vi "lpf.vi"(1 "Signals":waveform(dbl)[](array[waveform])) -> (0 "FIltered signals":waveform(dbl)[](array[waveform]))   [LabVIEW 2021]
uses:
  <vilib>/Analysis/3filter.llb/Filter Passband Type.ctl
  <vilib>/Analysis/3filter.llb/Butterworth Filter (DBL).vi
  <vilib>/Analysis/NI_AALBase.lvlib
panel:
  in  "Cutoff frequency, Hz":dbl=100.0
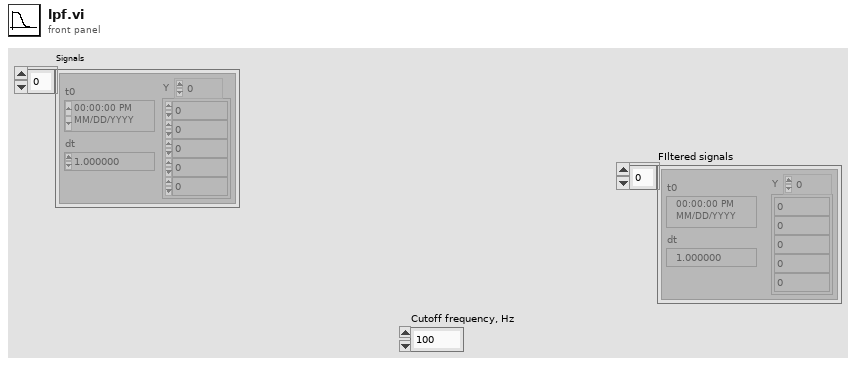
[diagram p1: front panel]
types:
  T1 = typedef "NI_AALBase.lvlib/Filter Passband Type.ctl" = enum32{"Lowpass", "Highpass", "Bandpass", "Bandstop"}
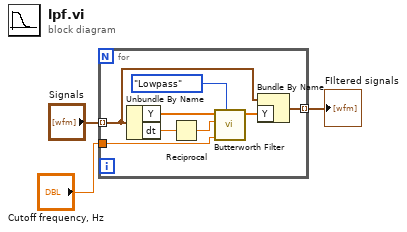
[diagram p0: block diagram]
diagram:
  n1 = for {
    tunnel: "Signals" -> [w6] mode=indexing
    tunnel: "Cutoff frequency, Hz" -> [w7]
    tunnel: [w4] -> w1 mode=indexing
    n2 = Unbundle By Name(w6) -> ("Y"=w11:dbl[], "dt"=w10:dbl)
    n3 = Reciprocal(x=w10) -> (1/x=w9:dbl)
    n4 = call-poly <vilib>:"Butterworth Filter.vi"("filter type"=Filter_Passband_Type."Lowpass", "low cutoff freq: fl"=w7, "sampling freq: fs"=w9, "X"=w11) -> ("Filtered X"=w5:dbl[])  [unwired: 4 in, 1 out]
    n5 = Bundle By Name(cluster=w6, "Y"=w5) -> (w4:waveform(dbl))
  }
  "FIltered signals" <- w1
